vi "AES Encryption Test.vi"() -> ()   [LabVIEW 2012]
doc: "Demonstrates operation of LabVIEW AES library."
uses:
  Advanced Encryption Standard (AES).lvlib
panel:
  out "Is Decrypted text identical?":bool
  out "milliseconds":u32
  out "Encrypted Text Out":string
  out "Decrypted Text Out":string
  in  "Plain Text In":string="The string you want to encrypt."
  in  "Password In":string="Very strong password here"
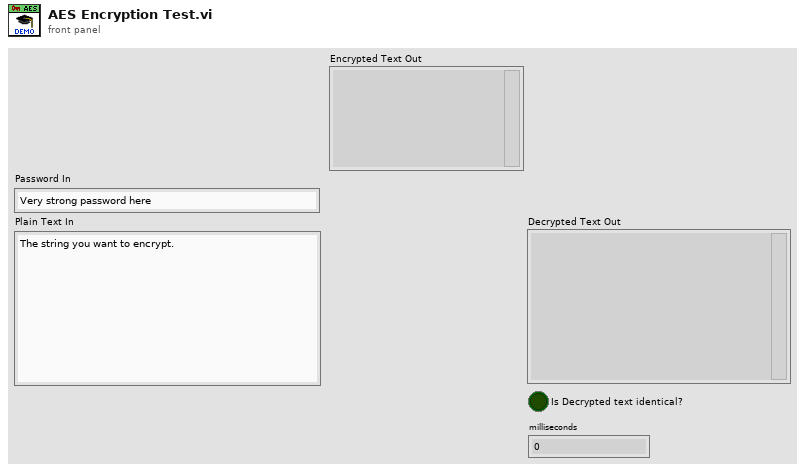
[diagram p1: front panel]
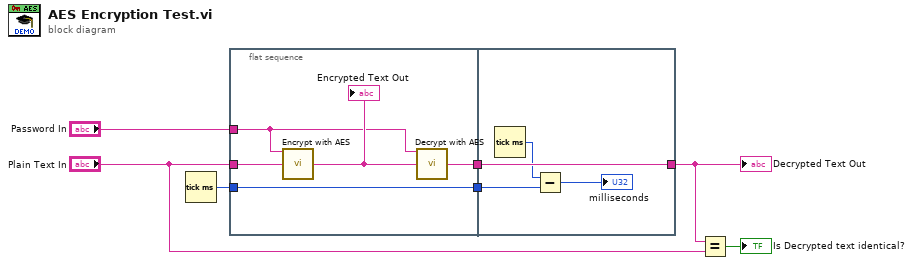
[diagram p0: block diagram]
diagram:
  n1 = Tick Count (ms)() -> (millisecond timer value=w4:u32)
  n2 = flat-sequence {
    tunnel: [w8] -> w7
    tunnel: "Plain Text In" -> [w11]
    tunnel: "Password In" -> [w9]
    tunnel: w4 -> [w12]
    tunnel: [w12] -> w6
    tunnel: [w16] -> w1
    tunnel: w7 -> [w16]
    tunnel: w6 -> [w14]
    frame #0 {
      n3 = call "Encrypt with AES.vi"("Password.In"=w9, "Plain Text In"=w11) -> ("Cyphered Text out"=w10:string)  [unwired: 12 in, 1 out]
      "Encrypted Text Out" <- w10
      n4 = call "Decrypt with AES.vi"("Password.In"=w9, "EncryptedText.In"=w10) -> ("DecryptedText.Out"=w8:string)  [unwired: 12 in, 1 out]
    }
    frame #1 {
      n5 = Tick Count (ms)() -> (millisecond timer value=w15:u32)
      n6 = Subtract(x=w15, y=w14) -> (x-y=→"milliseconds":u32)
    }
  }
  n7 = Equal?(x=w1, y="Plain Text In") -> (x = y?=→"Is Decrypted text identical?":bool)
  "Decrypted Text Out" <- w1
